vi "phythog.vi"() -> ()   [LabVIEW 2009]
panel:
  out "Numeric 3":dbl
  in  "Numeric 2":dbl
  in  "Numeric":dbl
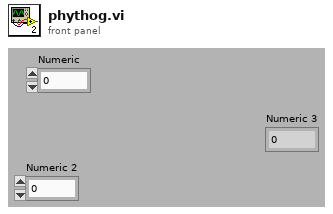
[diagram p1: front panel]
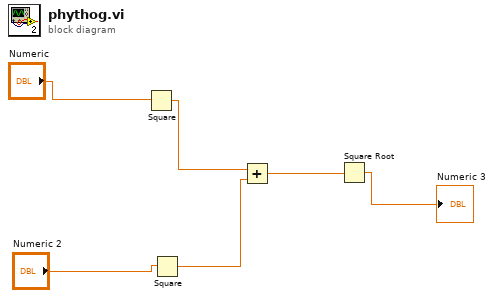
[diagram p0: block diagram]
diagram:
  n1 = Square(x="Numeric") -> (x^2=w4:dbl)
  n2 = Square(x="Numeric 2") -> (x^2=w3:dbl)
  n3 = Add(x=w4, y=w3) -> (x+y=w2:dbl)
  n4 = Square Root(x=w2) -> (sqrt(x)=→"Numeric 3":dbl)
